vi "zc_jd.vi"(0 "action":string, 1 "LabVIEW Web Service Request":refnum<class "Web Request.lvclass"> caption="LabVIEW Web服务请求", 2 "jddidian":string, 3 "sp_yijian":string, 4 "key":string, 5 "id":string, 7 "zc_luodi_num":string, 8 "sp_shuoming":string, 9 "jddanwei":string, 10 "zhriqi":string, 11 "jdren":string, 12 "jdlxfs":string, 13 "shuoming":string, 14 "lc_num":string) -> (15 "error":errorcluster)   [LabVIEW 2017]
uses:
  <vilib>/wsapi/Web Request.lvclass
panel:
  in  "error 3":errorcluster={"status"=TRUE, "code"=255, "source"="当前资产不是“领用”状态！"} caption="error"
  out "postdata":string caption="post数据"
  out "error out":errorcluster caption="错误输出"
  # "Web服务请求输入接线端用于调用“Web服务”选板的VI。除非不需要访问该选板，否则不要在连线板上删除这个输入接线端。"
  # "添加至连线板的每一个其他输入控件，在URL中对应于一个输入。如需在接线端模式输出（默认设置）下包含显示控件，则该显示控件必须与连线板相连。"
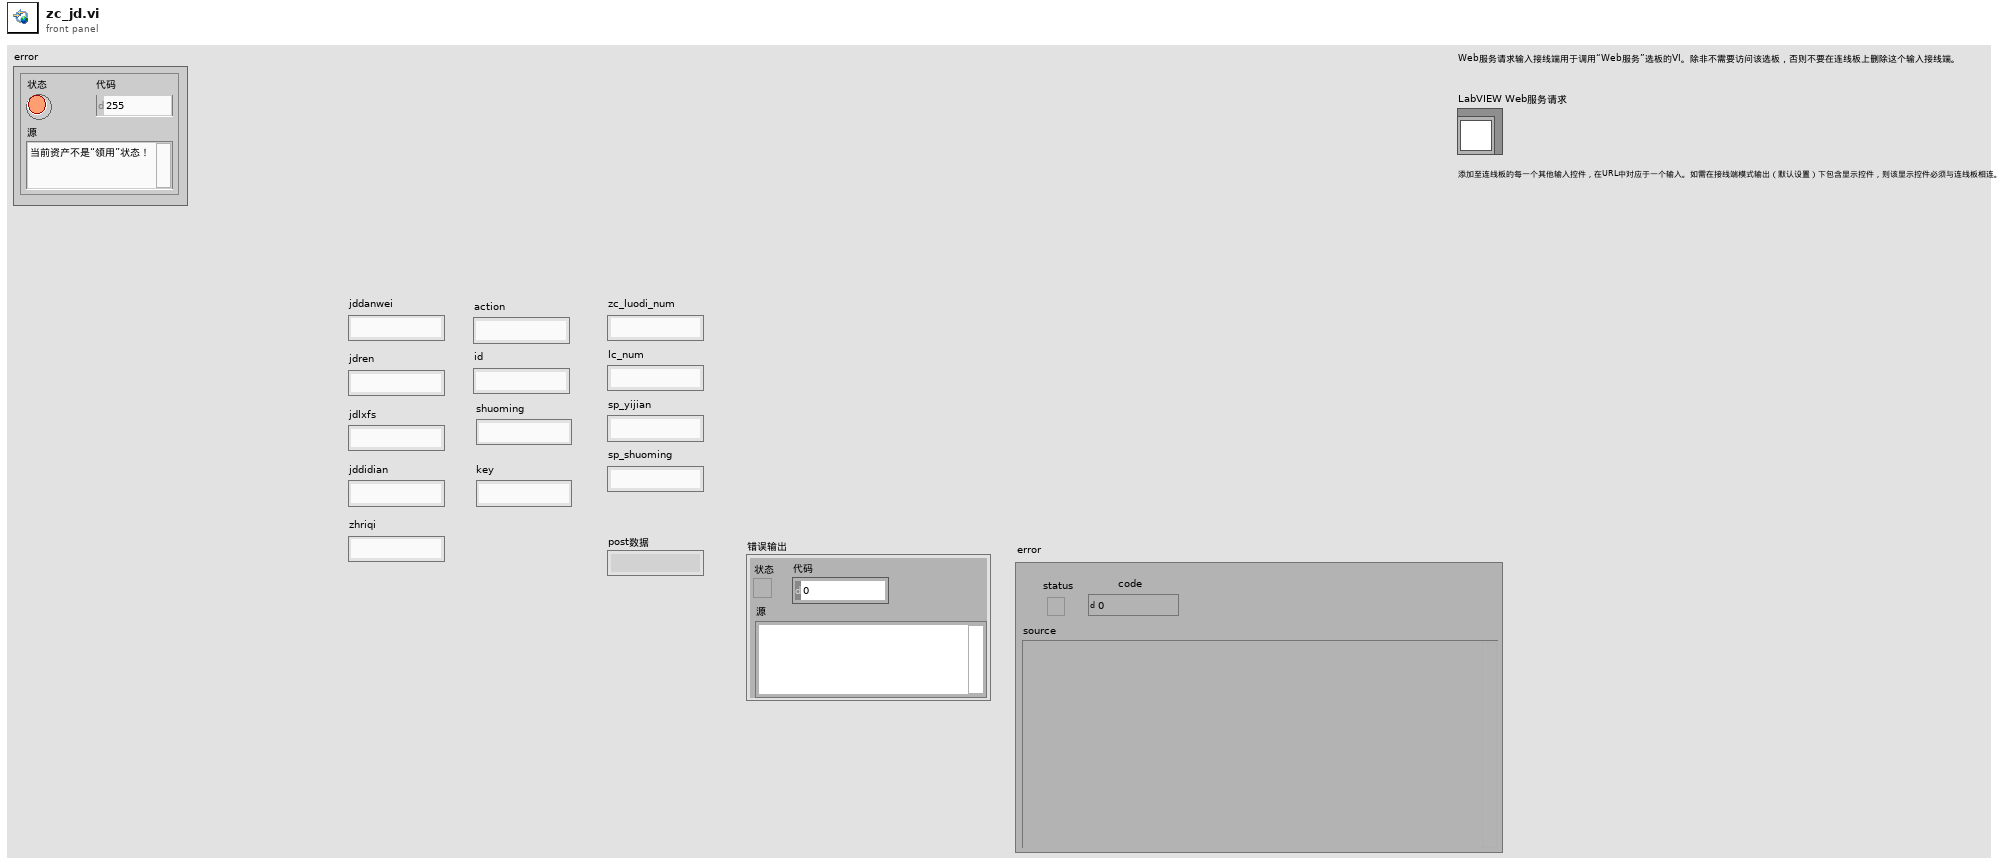
[diagram p1: front panel]
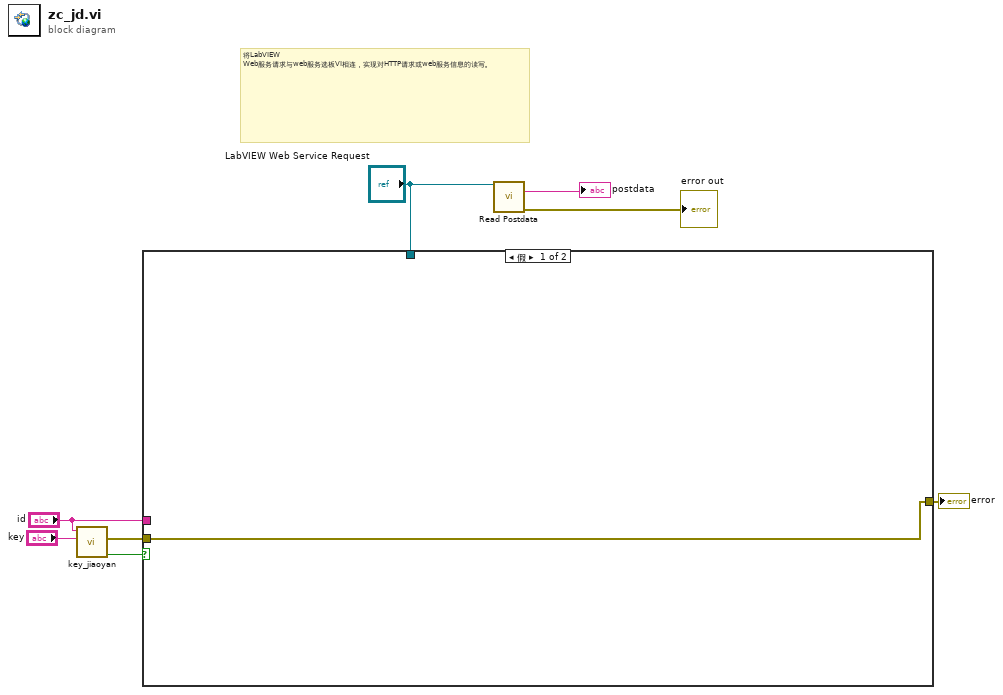
[diagram p0: block diagram]
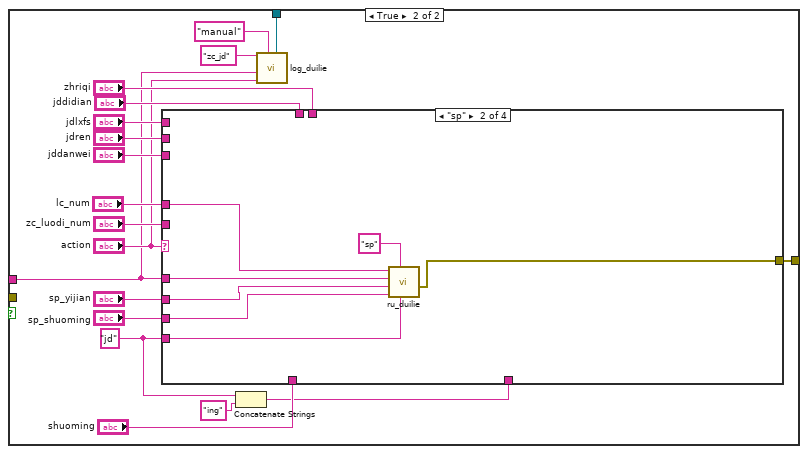
[diagram p2: hidden frame]
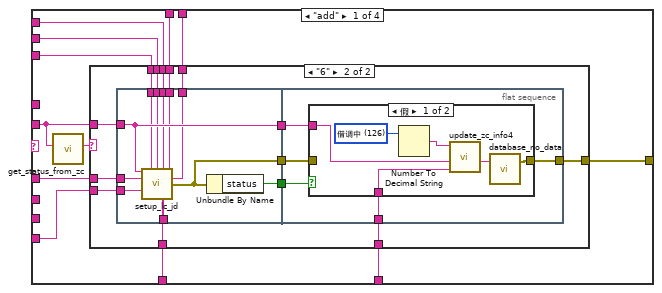
[diagram p3: hidden frame]
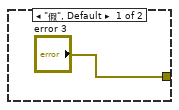
[diagram p4: hidden frame]
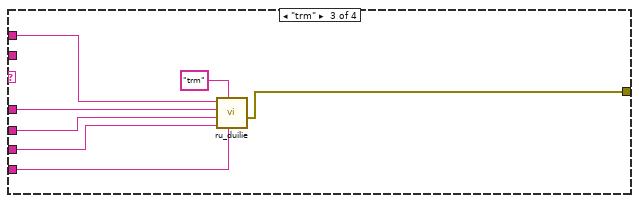
[diagram p6: hidden frame]
diagram:
  # "将LabVIEW Web服务请求与web服务选板VI相连，实现对HTTP请求或web服务信息的读写。"
  n1 = call "key_jiaoyan.vi"("key_client"="key", "gonghao"="id") -> ("jy"=w2:bool, "error"=w1:errorcluster)  [unwired: 8 in]
  n2 = case shown="假" w2 {
    tunnel: [w9 w23] -> w7
    tunnel: "LabVIEW Web Service Request" -> [_ w12]
    tunnel: "id" -> [_ w10]
    tunnel: w1 -> [w9 _]
    frame False {
    }
    frame True {
      w15 = "jd" ("yw")
      n3 = Concatenate Strings(w15, "ing" ("字符串")) -> (w21:string)
      n4 = case shown="\"sp\"" "action" {
        tunnel: w10 -> [w39 w84 w91 _]
        tunnel: "zc_luodi_num" -> [w30 _ _ _]
        tunnel: "sp_yijian" -> [_ w82 w89 _]
        tunnel: "sp_shuoming" -> [_ w81 w88 _]
        tunnel: "shuoming" -> [w40 _ _ _]
        tunnel: w15 -> [w38 w80 w87 _]
        tunnel: "lc_num" -> [_ w83 w90 _]
        tunnel: [w37 w79 w86 _] -> w23
        tunnel: w21 -> [w36 _ _ _]
        tunnel: "jddanwei" -> [w35 _ _ _]
        tunnel: "jdren" -> [w34 _ _ _]
        tunnel: "jdlxfs" -> [w33 _ _ _]
        tunnel: "jddidian" -> [w32 _ _ _]
        tunnel: "zhriqi" -> [w31 _ _ _]
        frame "add" {
          n5 = call "get_status_from_zc.vi"("zc_luodi_num"=w30) -> ("status"=w29:string)  [unwired: 9 in, 1 out]
          n6 = case shown="\"6\"" w29 {
            tunnel: w40 -> [_ w54]
            tunnel: w39 -> [_ w53]
            tunnel: w38 -> [_ w52]
            tunnel: ["error 3" w51] -> w37
            tunnel: w36 -> [_ w50]
            tunnel: w35 -> [_ w49]
            tunnel: w34 -> [_ w48]
            tunnel: w33 -> [_ w47]
            tunnel: w32 -> [_ w46]
            tunnel: w31 -> [_ w45]
            tunnel: w30 -> [_ w44]
            frame "假", Default {
            }
            frame "6" {
              n7 = flat-sequence {
                tunnel: w54 -> [w63]
                tunnel: w44 -> [w66]
                tunnel: w53 -> [w65]
                tunnel: w52 -> [w64]
                tunnel: [w66] -> w55
                tunnel: w49 -> [w62]
                tunnel: w48 -> [w61]
                tunnel: w47 -> [w60]
                tunnel: w46 -> [w59]
                tunnel: w45 -> [w58]
                tunnel: [w57] -> w43
                tunnel: [w56] -> w42
                tunnel: w55 -> [w69]
                tunnel: [w71] -> w51
                tunnel: w50 -> [w70]
                tunnel: w43 -> [w68]
                tunnel: w42 -> [w67]
                frame #0 {
                  n8 = call "setup_lc_jd.vi"("zc_luodi_num"=w66, "jddanwei"=w62, "jdren"=w61, "jdlxfs"=w60, "jddidian"=w59, "id"=w65, "zhriqi"=w58, "yw"=w64, "shuoming"=w63) -> ("error"=w56:errorcluster)  [unwired: 6 in]
                  n9 = Unbundle By Name(w56) -> ("status"=w57:bool)
                }
                frame #1 {
                  n10 = case shown="假" w68 {
                    tunnel: [w75 w78] -> w71
                    tunnel: w70 -> [w74 _]
                    tunnel: w69 -> [w72 _]
                    tunnel: w67 -> [_ w78]
                    frame False {
                      w73 = u8 126 items=["待验收"=1, "无需验收"=2, "验收不合格"=3, "待入库"=4, "入库"=5, "领用"=6, "借用"=7, "托管"=8, "接管"=9, "退出"=10, "出库在用"=11, "盘亏"=12, "出售"=13, "报废"=14, "领用中"=120, "退库中"=121, "借用中"=122, "归还中"=123, "转移中"=124, "调拨中"=125, "借调中"=126, "托管中"=127, "终止托管中"=128, "退出中"=129, "处置中"=130] ("状态选择器")
                      n11 = Number To Decimal String(number=w73) -> (decimal integer string=w76:string)  [unwired: 1 in]
                      n12 = call "update_zc_info4.vi"("ywxinxi"=w74, "number"=w72, "status"=w76) -> ("data_str"=w77:string)  [unwired: 8 in]
                      n13 = call "database_no_data.vi"("input"=w77) -> ("error"=w75:errorcluster)  [unwired: 2 in]
                    }
                    frame True {
                    }
                  }
                }
              }
            }
          }
        }
        frame "sp" {
          n14 = call "ru_duilie.vi"("yw"=w80, "name"="sp" ("元素"), "sp_shuoming"=w81, "sp_yijian"=w82, "id"=w84, "lc_num"=w83) -> ("error"=w79:errorcluster)  [unwired: 5 in]
        }
        frame "trm" {
          n15 = call "ru_duilie.vi"("yw"=w87, "name"="trm" ("元素"), "sp_shuoming"=w88, "sp_yijian"=w89, "id"=w91, "lc_num"=w90) -> ("error"=w86:errorcluster)  [unwired: 5 in]
        }
        frame Default {
        }
      }
      n16 = call "log_duilie.vi"("LabVIEW Web Service Request"=w12, "type"="manual", "action"="action", "user"=w10, "yw"="zc_jd") -> ()  [unwired: 7 in]
    }
  }
  "error" <- w7
  n17 = call <vilib>:"Read Postdata.vi"("LabVIEW Web Service Request"="LabVIEW Web Service Request") -> ("postdata"=→"postdata":string, "error out"=→"error out":errorcluster)  [unwired: 12 in, 1 out]
